vi "Read Measurement Data (Digital 1Chan).vi"(0 "VISA resource name":refnum<visa-resource-name>, 5 "Channel (1)":string="0001", 9 "Data Format (0 : Binary)":i32(ring) items=["Binary", "ASCII"], 11 "error in (no error)":errorcluster) -> (2 "Date Time":timestamp=timestamp(3345116400 s since 1904-01-01) format="%<%H:%M:%S%3u\n%x>T", 4 "VISA resource name out":refnum<visa-resource-name>, 6 "Channel":string, 8 "Data":u16, 10 "Data Status":i32(ring) items=["Normal", "Differential Input", "Skip", "Over", "Error", "Burnout", "Power Failure"], 13 "Alarm Status":i32[](array[ring]) items=["No Alarm", "High Limit Alarm (H)", "Low Limit Alarm (L)", "Difference High Limit Alarm (h)", "Difference Low Limit Alarm (l)", "High Limit on Rate-of-change Alarm (R)", "Low Limit on Rate-of-change Alarm (r)", "Delay High Limit Alarm (T)", "Delay Low Limit Alarm (t)"], 15 "error out":errorcluster)   [LabVIEW 2020, in "Yokogawa GX Series.lvlib"]
doc: "This VI reads the digital measurement data by ASCII or Binary."
uses:
  <instrlib>/Yokogawa GX Series/Yokogawa GX Series.lvlib
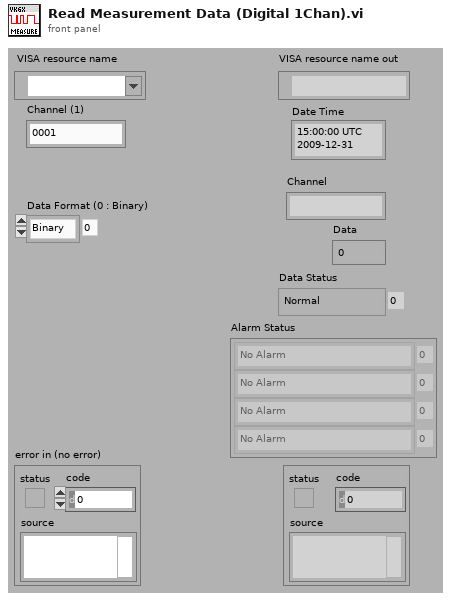
[diagram p1: front panel]
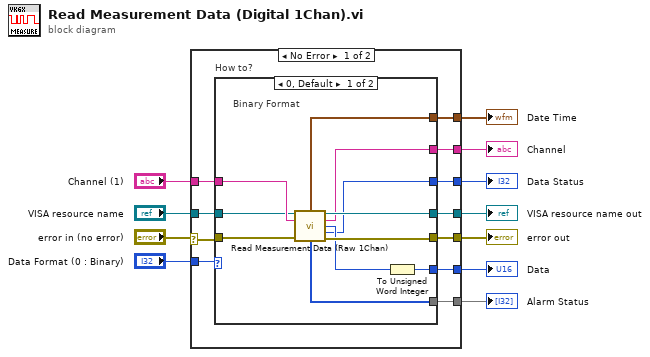
[diagram p0: block diagram]
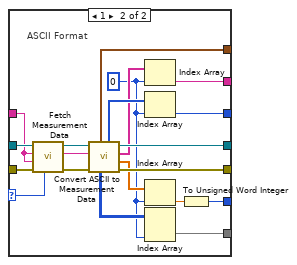
[diagram p2: hidden frame]
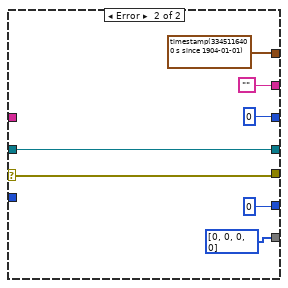
[diagram p3: hidden frame]
diagram:
  n1 = case shown="No Error" "error in (no error)" {
    selector: "error in (no error)" -> [w12 w59]
    tunnel: "VISA resource name" -> [w22 w60]
    tunnel: [w21 w60] -> w10
    tunnel: [w20 w59] -> w9
    tunnel: "Data Format (0 : Binary)" -> [w19 _]
    tunnel: [w18 timestamp(3345116400 s since 1904-01-01)] -> w7
    tunnel: [w17 ""] -> w6
    tunnel: [w16 u16 0] -> w5
    tunnel: [w15 i32[] [0, 0, 0, 0]] -> w4
    tunnel: [w14 0] -> w3
    tunnel: "Channel (1)" -> [w13 _]
    frame No Error {
      n2 = case "How to?" shown="0, Default" w19 {
        selector: w19 -> [_ w34]
        tunnel: w22 -> [w31 w53]
        tunnel: w12 -> [w30 w52]
        tunnel: [w29 w46] -> w21
        tunnel: [w28 w48] -> w20
        tunnel: w13 -> [w32 w45]
        tunnel: [w27 w47] -> w18
        tunnel: [w26 w42] -> w17
        tunnel: [w33 w38] -> w16
        tunnel: [w24 w40] -> w14
        tunnel: [w23 w39] -> w15
        frame 0, Default {
          # "Binary Format"
          n3 = call <instrlib>:"Read Measurement Data (Raw 1Chan).vi"("VISA resource name"=w31, "Channel (1)"=w32, "error in (no error)"=w30) -> ("Date Time"=w27:timestamp, "VISA resource name out"=w29:refnum<visa-resource-name>, "Channel"=w26:string, "Data"=w25:i32, "Data Status"=w24:i32, "Alarm Status"=w23:i32[], "error out"=w28:errorcluster)  [unwired: 6 out]
          n4 = To Unsigned Word Integer(number=w25) -> (unsigned 16bit integer=w33:u16)
        }
        frame 1 {
          w35 = 0
          # "ASCII Format"
          n5 = call <instrlib>:"Fetch Measurement Data.vi"("Data Format (0 : Binary)"=w34, "error in (no error)"=w52, "End Channel (1)"=w45, "Start Channel (1)"=w45, "VISA resource name"=w53) -> ("error out"=w49:errorcluster, "Measurement Data"=w50:string, "VISA resource name out"=w51:refnum<visa-resource-name>)  [unwired: 4 out]
          n6 = call <instrlib>:"Convert ASCII to Measurement Data.vi"("error in (no error)"=w49, "Measurement ASCII Data (\"\")"=w50, "VISA resource name"=w51) -> ("error out"=w48:errorcluster, "Data"=w44:dbl[], "Channel"=w36:string[], "VISA resource name out"=w46:refnum<visa-resource-name>, "Data Status"=w43:i32[], "Alarm Status"=w37:i32[][], "Date Time"=w47:timestamp)  [unwired: 2 out]
          n7 = Index Array(array=w36, index=w35) -> (element=w42:string)
          n8 = Index Array(array=w43, index=w35) -> (element=w40:i32)
          n9 = Index Array(array=w44, index=w35) -> (element=w41:dbl)
          n10 = Index Array(array=w37, index (col)=w35) -> (element=w39:i32[])  [unwired: 1 in]
          n11 = To Unsigned Word Integer(number=w41) -> (unsigned 16bit integer=w38:u16)
        }
      }
    }
    frame Error {
    }
  }
  "error out" <- w9
  "VISA resource name out" <- w10
  "Channel" <- w6
  "Alarm Status" <- w4
  "Date Time" <- w7
  "Data" <- w5
  "Data Status" <- w3
